vi "FrequencyCounter CountChange Event Example.vi"() -> ()   [LabVIEW 2012, in "Phidget Frequency Counter.lvlib"]
uses:
  <instrlib>/Phidgets/Phidget Frequency Counter/Phidget Frequency Counter.lvlib
  <instrlib>/Phidgets/Phidget Frequency Counter/Public/FrequencyCounterStart.vi
  <instrlib>/Phidgets/Phidget Frequency Counter/Public/FrequencyCounterClose.vi
  <instrlib>/Phidgets/Phidget Common/Phidget Common.lvlib
panel:
  out "TimeChange (ms)":dbl caption="TimeChange"
  out "CountChange":u64
  in  "stop":bool
  out "Serial Number Return":i32
  in  "Device Info":T1={"Serial Number"=-1, "Channel"=0, "Port"=0}
  out "error out":errorcluster
  # "Be sure to use this stop button to stop the program.\nIf you use the \"Abort Execution\" button, you will\nneed to use PhidgetResetLibrary.vi or restart Labview \nin order for any Phidgets to work."
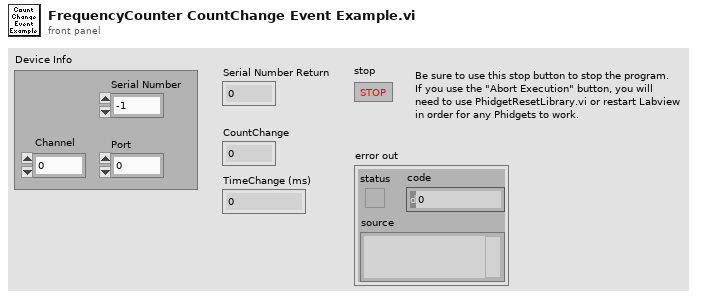
[diagram p1: front panel]
types:
  T1 = cluster{"Serial Number":i32, "Channel":i32, "Port":i32}
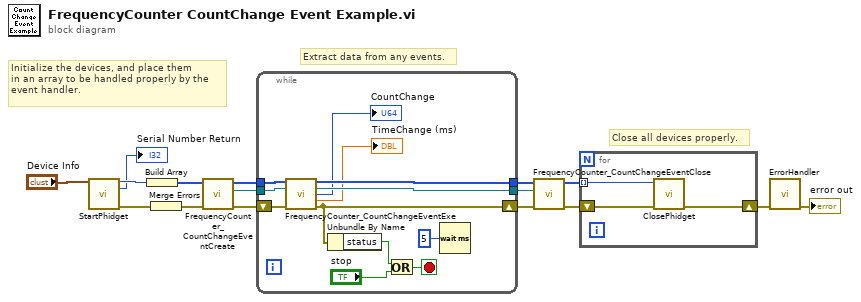
[diagram p0: block diagram]
diagram:
  # "Close all devices properly."
  # "Extract data from any events."
  # "Initialize the devices, and place them\nin an array to be handled properly by the\nevent handler."
  n1 = call-poly <instrlib>:"StartPhidget.vi"("Device Info"="Device Info") -> ("Phidget ID"=w7:u64, "Serial Number Return"=→"Serial Number Return":i32, "error out"=w2:errorcluster)  [unwired: 11 in, 1 out]
  n2 = Build Array(w7) -> (w16:u64[])
  n3 = Merge Errors(w2) -> (w9:errorcluster)
  n4 = call <instrlib>:"FrequencyCounter_CountChangeEventCreate.vi"("error in (no error)"=w9, "Devices In"=w16) -> ("error out"=w11:errorcluster, "Event Registration Refnum"=w4:refnum<event-registration>, "Devices Out"=w15:u64[])  [unwired: 7 in]
  n5 = while {
    tunnel: w15 -> [w28]
    tunnel: w4 -> [w23]
    tunnel: [w27] -> w3
    shift-right: [w22] -> w12
    shift-left: w11 -> [w26]
    tunnel: [w24] -> w5
    stop <- w21 stop-if-true
    n6 = call <instrlib>:"FrequencyCounter_CountChangeEventExe.vi"("Devices In"=w28, "Event Registration Refnum In"=w23, "error in (no error)"=w26) -> ("Devices Out"=w24:u64[], "Event Registration Refnum Out"=w27:refnum<event-registration>, "CountChange"=→"CountChange":u64, "TimeChange"=→"TimeChange (ms)":dbl, "error out"=w22:errorcluster)  [unwired: 5 in, 3 out]
    n7 = Unbundle By Name(w22) -> ("status"=w19:bool)
    n8 = Or(x=w19, y="stop") -> (x .or. y?=w21:bool)
    n9 = Wait (ms)(milliseconds to wait=u32 5) -> ()  [unwired: 1 out]
  }
  n10 = call <instrlib>:"FrequencyCounter_CountChangeEventClose.vi"("error in (no error)"=w12, "Event Registration Refnum In"=w3, "Devices In"=w5) -> ("error out"=w8:errorcluster, "Devices Out"=w6:u64[])  [unwired: 7 in]
  n11 = for {
    tunnel: w6 -> [w29] mode=indexing
    shift-right: [w31] -> w14
    shift-left: w8 -> [w30]
    n12 = call-poly <instrlib>:"ClosePhidget.vi"("error in"=w30, "Device In"=w29) -> ("error out"=w31:errorcluster)  [unwired: 9 in]
  }
  n13 = call <instrlib>:"ErrorHandler.vi"("error in"=w14) -> ("error out"=→"error out":errorcluster)  [unwired: 9 in, 1 out]
